vi "subGenerateDGMLExternal.vi"(7 "Expand?":bool, 9 "Nodes in in":T1, 10 "union in":T1, 11 "format string":string) -> (1 "Nodes out":T1, 2 "union out":T1)   [LabVIEW 2020, in "DefaultExtensions.lvlib" / "CGrapherDGML.lvclass"]
uses:
  CGrapherDGML.lvclass
  LabVIEWItem/CLabVIEWItem/ConnectionSet.ctl
  98aa7cab-ea86-498c-bf1b-cbfaad68de17.vi
  LabVIEWItem/CLabVIEWItem/CLabVIEWItem.lvclass
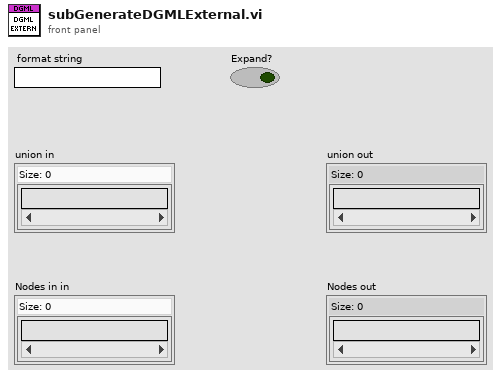
[diagram p1: front panel]
types:
  T1 = typedef "LabVIEWItem.lvlib/CLabVIEWItem.lvclass/ConnectionSet.ctl" = set{string}
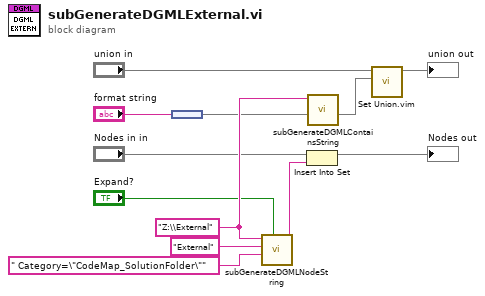
[diagram p0: block diagram]
diagram:
  w11 = "Z:\\External" ("format string")
  n1 = node("format string") -> (w7:set{string})
  n2 = call "subGenerateDGMLNodeString.vi"("Expand?"="Expand?", "Code schema"=" Category=\"CodeMap_SolutionFolder\"" ("format string"), "Label"="External" ("format string"), "Id"=w11) -> ("Node string"=w6:string)  [unwired: 7 in]
  n3 = Insert Into Set(10:w6, 11:"Nodes in in") -> (3:→"Nodes out":T1)  [unwired: 1 out]
  n4 = call "subGenerateDGMLContainsString.vi"("Contained"=w7, "Source"=w11) -> ("Links"=w10:T1)  [unwired: 9 in]
  n5 = call "Set Union.vim"("set 2"=w10, "set 1"="union in") -> ("union"=→"union out":T1)  [unwired: 9 in]
